vi "Ventus - Connect.vi"(4 "error in":errorcluster, 5 "Connect?":bool=TRUE, 6 "VISA Refnum in":refnum<visa-resource-name>="COM4") -> (0 "error out":errorcluster, 1 "Status":string, 2 "Ventus Controls":T1={"Ventus Power"=0.0, "Open Serial"=FALSE, "VISA Refnum"="ASRL4::INSTR"} caption="output cluster" {"Ventus Power" min=0.0 max=100.0 step=0.1 scale=0.0..100.0}, 3 "Ventus Laser Connected":bool=TRUE)   [LabVIEW 2020]
uses:
  _controls/Ventus Control.ctl
  <vilib>/Instr/_visa.llb/VISA Configure Serial Port (Instr).vi
panel:
  in  "Intf Inst Name":string="ASRL4::INSTR"
  in  "regular expression":string="COM4"
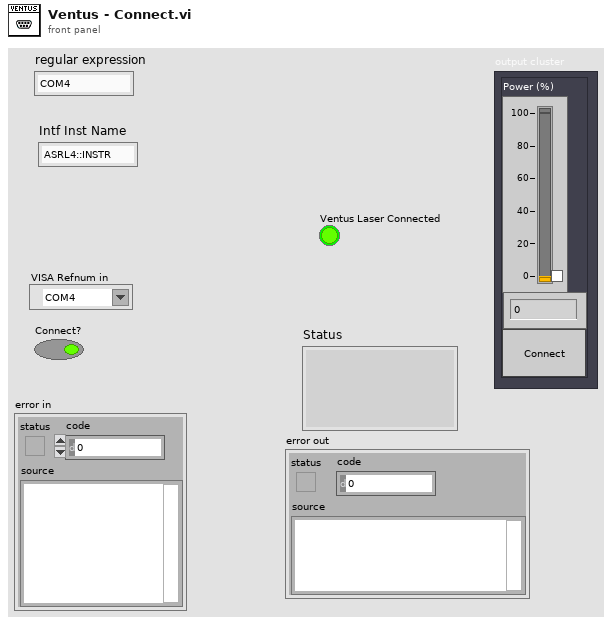
[diagram p1: front panel]
types:
  T1 = typedef "Ventus Control.ctl" = cluster{"Ventus Power":dbl, "Open Serial":bool, "VISA Refnum":refnum<visa-resource-name>}
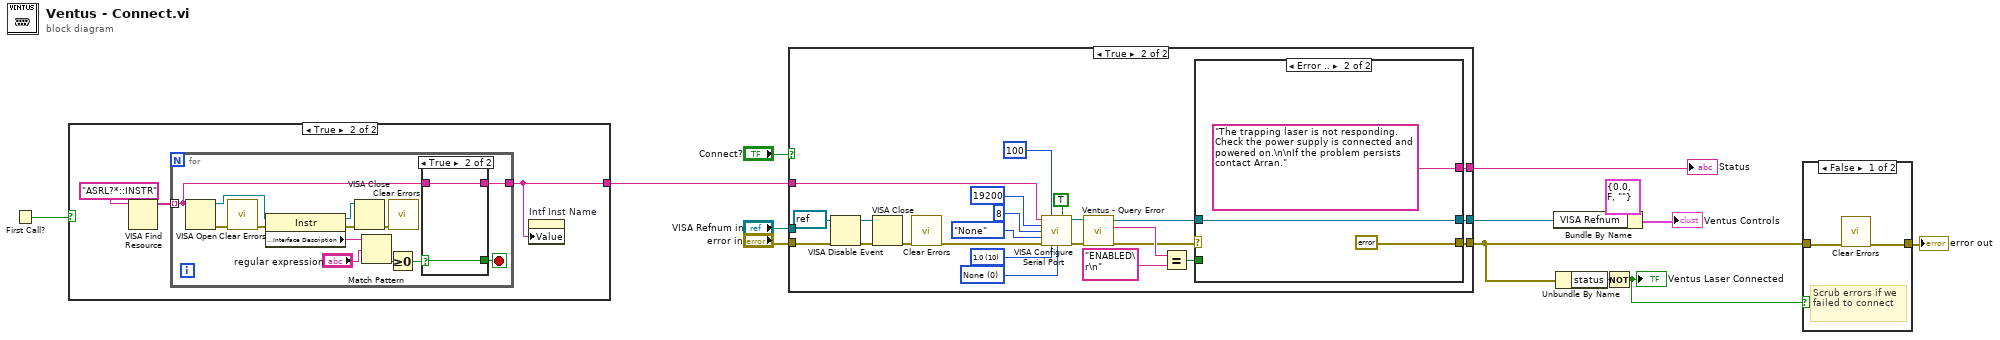
[diagram p0: block diagram]
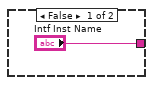
[diagram p3: hidden frame]
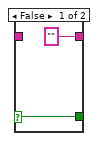
[diagram p4: hidden frame]
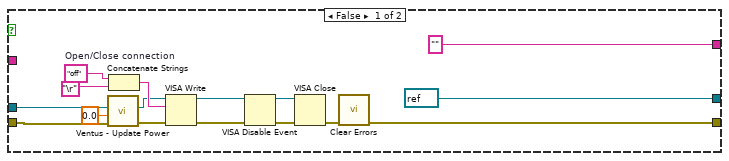
[diagram p5: hidden frame]
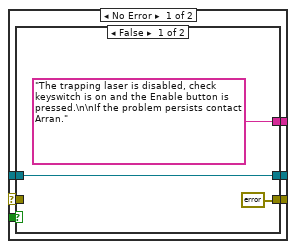
[diagram p6: hidden frame]
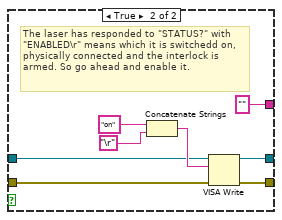
[diagram p7: hidden frame]
diagram:
  n1 = First Call?() -> (First Call?: T/F=w7:bool)
  n2 = case shown="True" w7 {
    tunnel: ["Intf Inst Name" w15] -> w10
    frame False {
    }
    frame True {
      n3 = VISA Find Resource(11:"ASRL?*::INSTR" ("expression (\"\")")) -> (3:w16:string[])  [unwired: 2 in, 2 out]
      n4 = for {
        tunnel: w16 -> [w19] mode=indexing
        tunnel: [w21] -> w15
        stop <- w22 stop-if-true
        n5 = VISA Open(VISA resource name=w19) -> (VISA resource name=w26:refnum<visa-resource-name>, error out=w29:errorcluster)  [unwired: 4 in]
        n6 = call <vilib>:"Clear Errors.vi"("error in (no error)"=w29) -> ("error out"=w25:errorcluster)  [unwired: 5 in, 1 out]
        n7 = property class="Instr"(reference=w26, error in=w25) -> (reference out=w30:refnum<visa-resource-name>, error out=w28:errorcluster, "Interface Information:Interface Description"=w23:string)
        n8 = VISA Close(VISA resource name=w30, error in (no error)=w28) -> (error out=w20:errorcluster)
        n9 = Match Pattern(string=w23, regular expression="regular expression") -> (offset past match=w18:i32)  [unwired: 1 in, 3 out]
        n10 = Greater Or Equal To 0?(x=w18) -> (x >= 0?=w24:bool)
        n11 = call <vilib>:"Clear Errors.vi"("error in (no error)"=w20) -> ()  [unwired: 5 in, 2 out]
        n12 = case shown="True" w24 {
          selector: w24 -> [w32 w34]
          tunnel: w19 -> [_ w33]
          tunnel: [w32 w34] -> w22
          tunnel: ["" ("Intf Inst Name") w33] -> w21
          frame False {
          }
          frame True {
          }
        }
      }
      n13 = property on="Intf Inst Name" class="Str"("Value"=w15) -> ()  [unwired: 2 in, 2 out]
    }
  }
  n14 = case shown="True" "Connect?" {
    tunnel: w10 -> [_ w59]
    tunnel: [w43 w73] -> w2
    tunnel: "error in" -> [w37 w72]
    tunnel: "VISA Refnum in" -> [w38 _]
    tunnel: [refnum<visa-resource-name> refnum ("VISA Refnum out") w63] -> w4
    tunnel: ["" w60] -> w8
    frame False {
      w47 = "off"  # Open/Close connection
      n15 = call "Ventus - Update Power.vi"("error in (no error)"=w37, "Power (%)"=0.0, "VISA resource name"=w38) -> ("error out"=w35:errorcluster, "VISA resource name out"=w36:refnum<visa-resource-name>)  [unwired: 3 in]
      n16 = Concatenate Strings(w47, "\r") -> (w45:string)
      n17 = VISA Write(VISA resource name=w36, write buffer=w45, error in (no error)=w35) -> (VISA resource name out=w44:refnum<visa-resource-name>, error out=w42:errorcluster)  [unwired: 1 out]
      n18 = VISA Disable Event(8:w42, 11:w44) -> (0:w48:errorcluster, 3:w50:refnum<visa-resource-name>)  [unwired: 2 in]
      n19 = VISA Close(VISA resource name=w50, error in (no error)=w48) -> (error out=w49:errorcluster)
      n20 = call <vilib>:"Clear Errors.vi"("error in (no error)"=w49) -> ("error out"=w43:errorcluster)  [unwired: 5 in, 1 out]
    }
    frame True {
      w71 = u16 0 items=["None", "XON/XOFF", "RTS/CTS", "XON/XOFF & RTS/CTS", "DTR/DSR", "XON/XOFF & DTR/DSR"] ("flow control (0:none)")
      w70 = u16 10 items=["1.0"=10, "1.5"=15, "2.0"=20] ("Stop Bits")
      n21 = VISA Disable Event(8:w72, 11:refnum<visa-resource-name> refnum ("VISA resource name")) -> (0:w65:errorcluster, 3:w67:refnum<visa-resource-name>)  [unwired: 2 in]
      n22 = VISA Close(VISA resource name=w67, error in (no error)=w65) -> (error out=w66:errorcluster)
      n23 = call <vilib>:"Clear Errors.vi"("error in (no error)"=w66) -> ("error out"=w74:errorcluster)  [unwired: 5 in, 1 out]
      n24 = call-poly "VISA Configure Serial Port"("VISA resource name"=w59, "timeout (10sec)"=u32 100, "Enable Termination\nChar (T)"=TRUE ("Enable Termination\nChar (T)"), "baud rate (9600)"=u32 19200, "data bits (8)"=u16 8 ("Data Bits"), "parity (0:none)"=enum16{"None", "Odd", "Even", "Mark", "Space"}."None" ("Parity"), "error in (no error)"=w74, "stop bits (10: 1 bit)"=w70, "flow control (0:none)"=w71) -> ("VISA resource name out"=w54:refnum<visa-resource-name>, "error out"=w53:errorcluster)  [unwired: 5 in]
      n25 = call "Ventus - Query Error.vi"("error in (no error)"=w53, "VISA Refnum in"=w54) -> ("error out"=w55:errorcluster, "Error Status"=w58:string, "VISA Refnum out"=w61:refnum<visa-resource-name>)  [unwired: 7 in]
      n26 = Equal?(x=w58, y="ENABLED\r\n") -> (x = y?=w56:bool)
      n27 = case shown="Error .." w55 {
        selector: w55 -> [w75 _]
        tunnel: [w80 errorcluster {"status"=TRUE, "code"=0, "source"=""} ("error constant")] -> w73
        tunnel: [w79 w93] -> w63
        tunnel: w61 -> [w78 w93]
        tunnel: [w77 "The trapping laser is not responding. Check the power supply is connected and powered on.\n\nIf the problem persists contact Arran."] -> w60
        tunnel: w56 -> [w76 _]
        frame No Error {
          n28 = case shown="False" w76 {
            tunnel: [errorcluster {"status"=TRUE, "code"=0, "source"=""} ("error constant") w90] -> w80
            tunnel: [w83 w88] -> w79
            tunnel: w78 -> [w83 w86]
            tunnel: w75 -> [_ w85]
            tunnel: ["The trapping laser is disabled, check keyswitch is on and the Enable button is pressed.\n\nIf the problem persists contact Arran." ""] -> w77
            frame False {
            }
            frame True {
              # "The laser has responded to \"STATUS?\" with \"ENABLED\\r\" means which it is switchedd on, physically connected and the interlock is armed. So go ahead and enable it."
              n29 = Concatenate Strings("on", "\r") -> (w89:string)
              n30 = VISA Write(VISA resource name=w86, write buffer=w89, error in (no error)=w85) -> (VISA resource name out=w88:refnum<visa-resource-name>, error out=w90:errorcluster)  [unwired: 1 out]
            }
          }
        }
        frame Error {
        }
      }
    }
  }
  "Status" <- w8
  n31 = Bundle By Name(cluster=T1 {"Ventus Power"=0.0, "Open Serial"=FALSE, "VISA Refnum"=""} ("Manlight Controls"), "VISA Refnum"=w4) -> (→"Ventus Controls":T1)
  n32 = Unbundle By Name(w2) -> ("status"=w11:bool)
  n33 = Not(x=w11) -> (.not. x?=w3:bool)
  "Ventus Laser Connected" <- w3
  n34 = case shown="False" w3 {
    tunnel: w2 -> [w96 w97]
    tunnel: [w95 w97] -> w1
    frame False {
      # "Scrub errors if we failed to connect"
      n35 = call <vilib>:"Clear Errors.vi"("error in (no error)"=w96) -> ("error out"=w95:errorcluster)  [unwired: 5 in, 1 out]
    }
    frame True {
    }
  }
  "error out" <- w1
